vi "Hydrosonic_Manual.vi"() -> ()   [LabVIEW 2011]
panel:
  out "Array":u32[](array[numeric])
  in  "Mode":T1(ring)
  out "Tranducer Value":dbl format="%.2f"
  out "Transducer Error Info":string
  in  "Set Tranducer Value":T2(ring)
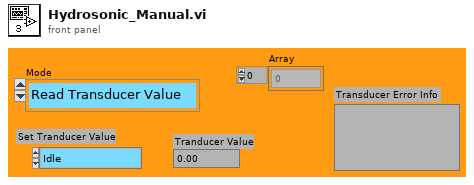
[diagram p1: front panel]
types:
  T1 = enum16{"Read Transducer Value", "Set Transducer value"}
  T2 = enum16{"Idle", "Pump out", "Pump in", "0", "14", "29", "43", "57", "71", "86", "100"}
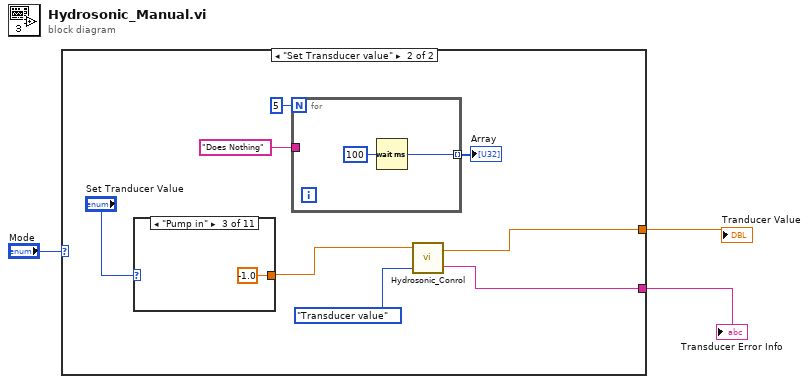
[diagram p0: block diagram]
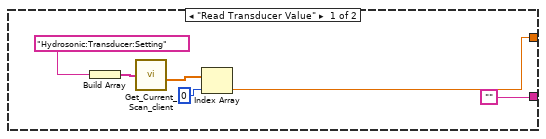
[diagram p2: hidden frame]
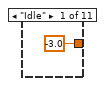
[diagram p3: hidden frame]
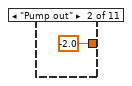
[diagram p4: hidden frame]
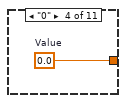
[diagram p5: hidden frame]
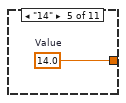
[diagram p6: hidden frame]
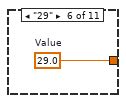
[diagram p7: hidden frame]
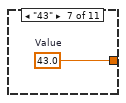
[diagram p8: hidden frame]
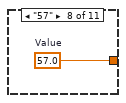
[diagram p9: hidden frame]
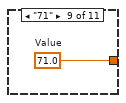
[diagram p10: hidden frame]
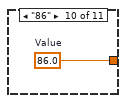
[diagram p11: hidden frame]
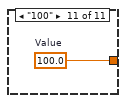
[diagram p12: hidden frame]
diagram:
  n1 = case shown="\"Set Transducer value\"" "Mode" {
    tunnel: [w4 w14] -> w3
    tunnel: ["" w13] -> w2
    frame "Read Transducer Value" {
      n2 = Build Array("Hydrosonic:Transducer:Setting") -> (w8:string[])
      n3 = call "Get_Current_Scan_client.vi"("ADAM Ch Names"=w8) -> ("Numerical Values"=w7:dbl[])  [unwired: 1 in, 2 out]
      n4 = Index Array(array=w7, index=0) -> (element=w4:dbl)
    }
    frame "Set Transducer value" {
      n5 = case shown="\"Pump in\"" "Set Tranducer Value" {
        tunnel: [-3.0 ("Value") -2.0 ("Value") -1.0 ("Value") w23 w24 w25 w26 w27 w28 w29 w30] -> w15
        frame "Idle" {
        }
        frame "Pump out" {
        }
        frame "Pump in" {
        }
        frame "0" {
          w23 = 0.0  # Value
        }
        frame "14" {
          w24 = 14.0  # Value
        }
        frame "29" {
          w25 = 29.0  # Value
        }
        frame "43" {
          w26 = 43.0  # Value
        }
        frame "57" {
          w27 = 57.0  # Value
        }
        frame "71" {
          w28 = 71.0  # Value
        }
        frame "86" {
          w29 = 86.0  # Value
        }
        frame "100" {
          w30 = 100.0  # Value
        }
      }
      n6 = for {
        N: 5 -> [_]
        tunnel: "Does Nothing" -> [_]
        tunnel: [w18] -> w10 mode=indexing
        n7 = Wait (ms)(milliseconds to wait=u32 100) -> (millisecond timer value=w18:u32)
      }
      "Array" <- w10
      n8 = call "Hydrosonic_Conrol.vi"("Input Mode"=enum16{"Desired Frequency", "Transducer value"}."Transducer value", "Desired Value"=w15) -> ("Error Info"=w13:string, "Set output"=w14:dbl)  [unwired: 2 in]
    }
  }
  "Transducer Error Info" <- w2
  "Tranducer Value" <- w3
